vi "Get Available Column Headers.vi"(8 "error in (no error)":errorcluster) -> (0 "error out":errorcluster, 3 "Available Column Headers":string[](array[string]))   [LabVIEW 2016, in "Assert API Components.lvlib" / "Assert Display.lvlib" / "Main Display.lvlib" / "Main Display.lvclass"]
uses:
  Main Display.lvclass
  <vilib>/Utility/config.llb/Read Key (String).vi
  <vilib>/Utility/config.llb/NI_LVConfig.lvlib
  Assert API Components/Assert API Components.lvlib
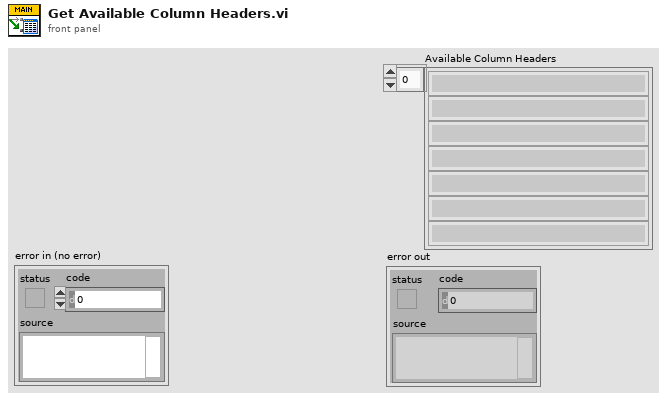
[diagram p1: front panel]
types:
  T1 = typedef "NI_LVConfig.lvlib/Config Data RefNum.ctl" = refnum<k1>
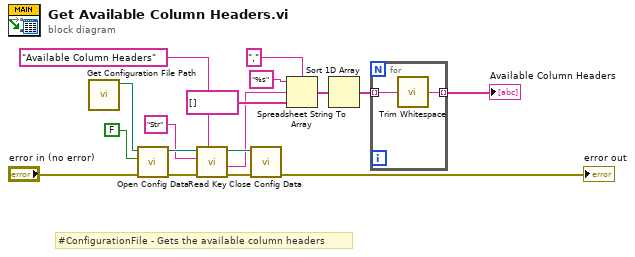
[diagram p0: block diagram]
diagram:
  # "#ConfigurationFile - Gets the available column headers"
  n1 = call "Get Configuration File Path.vi"() -> ("Configuration File Path"=w13:path)  [unwired: 11 in]
  n2 = call <vilib>:"Open Config Data.vi"("error in (no error)"="error in (no error)", "create file if necessary (T)"=FALSE, "configuration file path"=w13) -> ("error out"=w17:errorcluster, "refnum"=w15:T1)  [unwired: 6 in, 1 out]
  n3 = call-poly <vilib>:"Read Key.vi"("section"="Available Column Headers" ("key"), "error in (no error)"=w17, "key"="Str", "refnum"=w15) -> ("error out"=w16:errorcluster, "value"=w4:string, "refnum out"=w14:T1)  [unwired: 4 in, 1 out]
  n4 = call <vilib>:"Close Config Data.vi"("error in (no error)"=w16, "refnum"=w14) -> ("error out"=→"error out":errorcluster)  [unwired: 8 in, 1 out]
  n5 = Spreadsheet String To Array(delimiter (Tab)=",", format string="%s", spreadsheet string=w4, array type (2D Dbl)=string[] []) -> (array=w6:string[])
  n6 = Sort 1D Array(array=w6) -> (sorted array=w2:string[])
  n7 = for {
    tunnel: w2 -> [w19] mode=indexing
    tunnel: [w18] -> w1 mode=indexing
    n8 = call <vilib>:"Trim Whitespace.vi"("string"=w19) -> ("trimmed string"=w18:string)  [unwired: 1 in]
  }
  "Available Column Headers" <- w1
